vi "GetColor.vi"(8 "error in (no error)":errorcluster, 11 "ColorHSL in":refnum<class "ColorHSV.lvclass">) -> (0 "error out":errorcluster, 2 "Color":u32(colorbox), 3 "ColorHSL out":refnum<class "ColorHSV.lvclass">)   [LabVIEW 2021, in "Picture2D.lvlib" / "ColorHSV.lvclass"]
uses:
  ColorHSV.lvclass
  Color/Color.lvclass
  ColorHSV.lvclass/ColorHSV.ctl
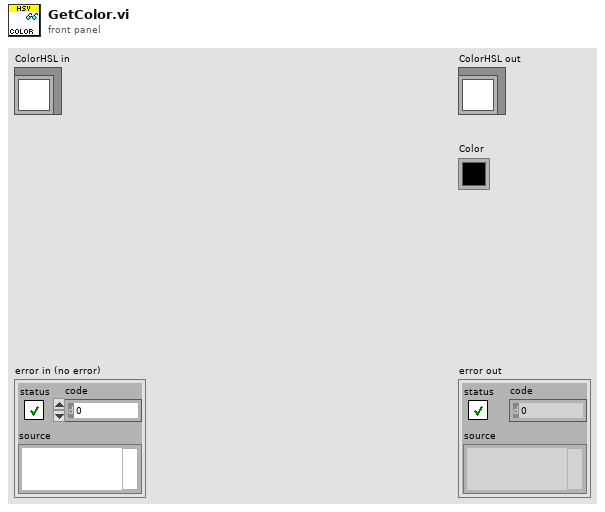
[diagram p1: front panel]
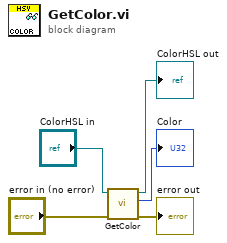
[diagram p0: block diagram]
diagram:
  n1 = call-parent "GetColor.vi"("error in (no error)"="error in (no error)", "Color in"="ColorHSL in") -> ("error out"=→"error out":errorcluster, "Color"=→"Color":u32, "Color out"=→"ColorHSL out":refnum<class "ColorHSV.lvclass">)  [unwired: 7 in]
